vi "Working With Arrays.vi"() -> ()   [LabVIEW 2016]
uses:
  API/JSON Document Class/json insert/json Insert - String Path.vi
  API/JSON Document Class/json parse/poly instances/json Parse U64 Array - string path.vi
  API/JSON Document Class/json parse/poly instances/json Parse I32 Array - string path.vi
  API/JSON Document Class/json to string/json To Minimized String - string path.vi
  API/JSON Document Class/JSON Document.lvclass
panel:
  out "I32 defaulted indices":i32[](array[numeric])
  out "I32 value":i32[](array[numeric])
  out "U64 defaulted indices":i32[](array[numeric])
  out "U64 value":u64[](array[numeric])
  out "json string":string
  # "[\n10,\n12,\n8,\n-1,\n2000000000000000000\n]"
  # "The special path \"/-\" allows us to easily\nbuild arrays."
  # "When the array is read as a U64 array, the value\n\"-1\" at index 3 is defaulted"
  # "When the array is read as an I32 array, the value\nat index 4 is too big for an I32 and is defaulted."
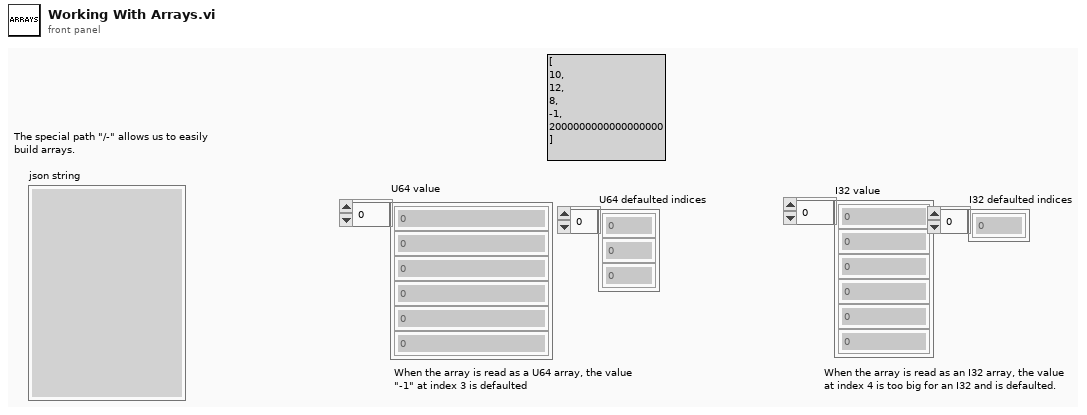
[diagram p1: front panel]
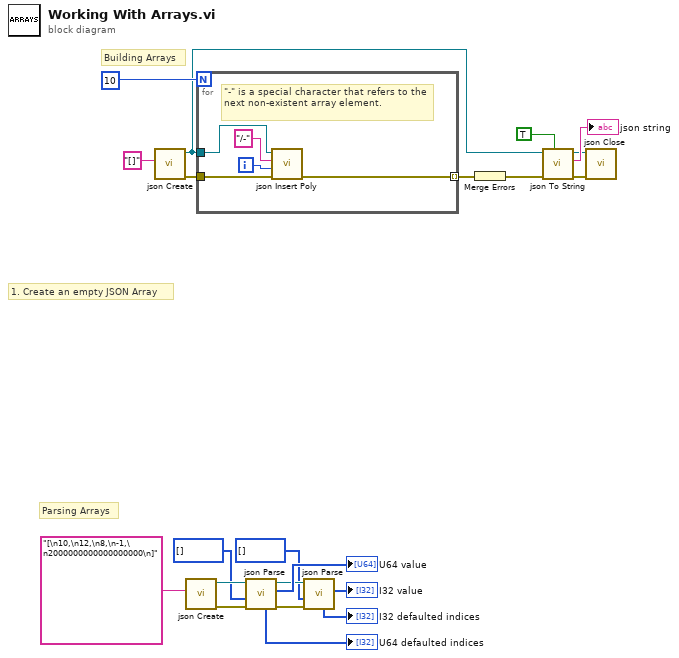
[diagram p0: block diagram]
diagram:
  # "1. Create an empty JSON Array"
  # "Parsing Arrays"
  # "Building Arrays"
  n1 = call "json Create.vi"("JSON String"="[]") -> ("error out"=w18:errorcluster, "JSON Document out"=w1:refnum<class "JSON Document.lvclass">)  [unwired: 9 in]
  n2 = call "json Create.vi"("JSON String"="[\n10,\n12,\n8,\n-1,\n2000000000000000000\n]") -> ("error out"=w10:errorcluster, "JSON Document out"=w11:refnum<class "JSON Document.lvclass">)  [unwired: 9 in]
  n3 = for {
    N: 10 -> [_]
    tunnel: w1 -> [w26]
    tunnel: [w24] -> w20 mode=indexing
    tunnel: w18 -> [w23]
    i -> [w25]
    # "\"-\" is a special character that refers to the next non-existent array element."
    n4 = call-poly "json Insert Poly.vi"("error in (no error)"=w23, "anything"=w25, "path"="/-", "JSON Document in"=w26) -> ("error out"=w24:errorcluster)  [unwired: 5 in, 2 out]
  }
  n5 = call-poly "json Parse.vi"("error in (no error)"=w10, "default"=u64[] [], "JSON Document in"=w11) -> ("error out"=w5:errorcluster, "value"=→"U64 value":u64[], "JSON Document out"=w6:refnum<class "JSON Document.lvclass">, "defaulted indices"=→"U64 defaulted indices":i32[])  [unwired: 4 in, 1 out]
  n6 = call-poly "json Parse.vi"("error in (no error)"=w5, "default"=i32[] [], "JSON Document in"=w6) -> ("value"=→"I32 value":i32[], "defaulted indices"=→"I32 defaulted indices":i32[])  [unwired: 4 in, 3 out]
  n7 = Merge Errors(w20) -> (w19:errorcluster)
  n8 = call-poly "json To String.vi"("pretty print?"=TRUE, "error in (no error)"=w19, "JSON Document in"=w1) -> ("error out"=w13:errorcluster, "json string"=→"json string":string, "JSON Document out"=w14:refnum<class "JSON Document.lvclass">)  [unwired: 6 in]
  n9 = call "json Close.vi"("error in (no error)"=w13, "JSON Document in"=w14) -> ()  [unwired: 9 in, 1 out]
